vi "MATLAB_SVD.vi"(11 "2IQ":csg[][](array[numeric])) -> (1 "V":cdb[][](array[numeric]), 3 "U":cdb[][](array[numeric]), 5 "Diag":dbl[](array[numeric]))   [LabVIEW 2022 SP3]
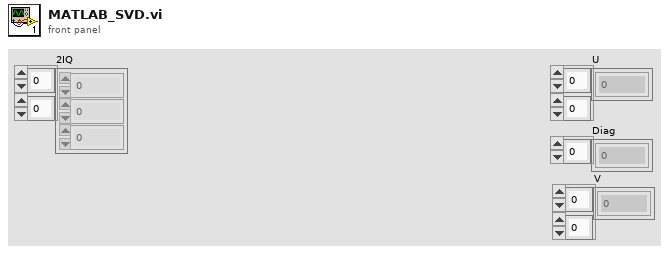
[diagram p1: front panel]
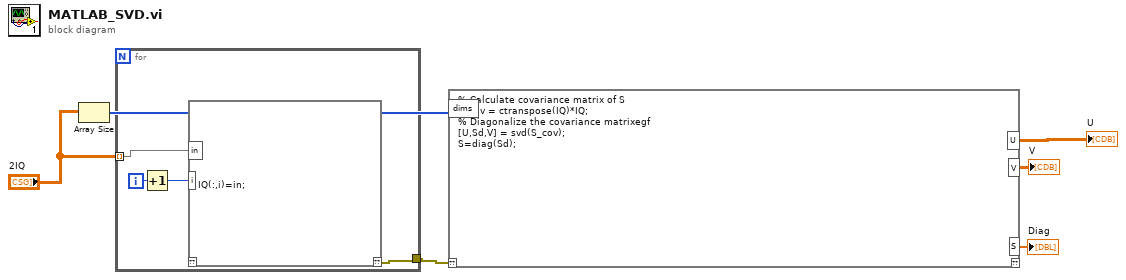
[diagram p0: block diagram]
diagram:
  n1 = Array Size(array="2IQ") -> (size(s)=w4:i32[])
  n2 = for {
    tunnel: "2IQ" -> [w7] mode=indexing
    tunnel: [w8] -> w1
    i -> [w10]
    n3 = Increment(x=w10) -> (x+1=w9:i32)
    n4 = script code="IQ(:,i)=in;"("in"=w7, "i"=w9) -> ("??"=w8:errorcluster)  [unwired: 1 in]
  }
  n5 = script code="% Calculate covariance matrix of S\nS_cov = ctranspose(IQ)*IQ;\n% Diagonalize the covariance matrixegf\n[U,Sd,V] = svd(S_cov);\nS=diag(Sd);"("??"=w1, "dims"=w4) -> ("U"=→"U":cdb[][], "S"=→"Diag":dbl[], "V"=→"V":cdb[][])  [unwired: 1 out]
